vi "RTP_RTSP - Parse RTP header.vi"(7 "RTP Packet":string) -> (8 "RTP Header":T1)   [LabVIEW 2014]
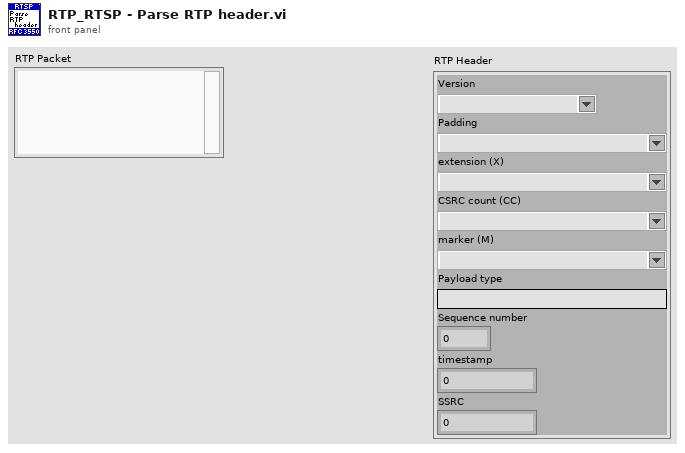
[diagram p1: front panel]
types:
  T1 = cluster{"Version":string, "Padding":string, "extension (X)":string, "CSRC count (CC)":string, "marker (M)":string, "Payload type":string, "Sequence number":u32, "timestamp":u32, "SSRC":u32}
  T2 = cluster{string, string, string, string, string, string, u32, u32, u32}
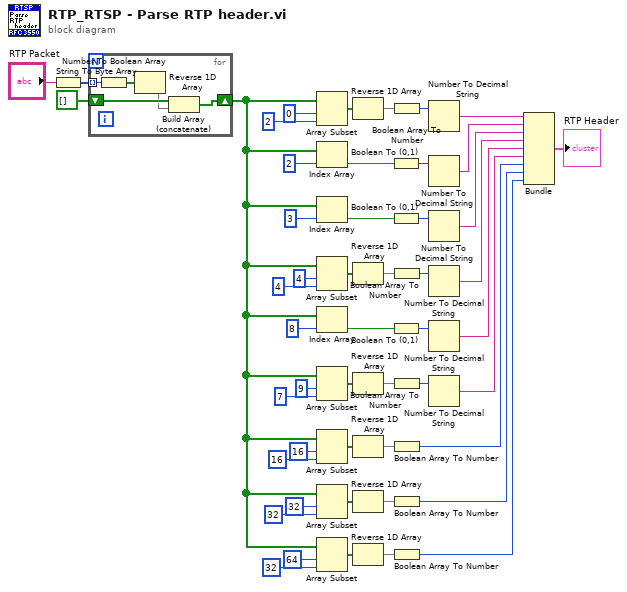
[diagram p0: block diagram]
diagram:
  n1 = String To Byte Array(string="RTP Packet") -> (unsigned byte array=w48:u8[])
  n2 = for {
    tunnel: w48 -> [w55] mode=indexing
    shift-right: [w52] -> w11
    shift-left: bool[] [] -> [w54]
    n3 = Number To Boolean Array(number=w55) -> (Boolean array=w53:bool[])
    n4 = Reverse 1D Array(array=w53) -> (reversed array=w51:bool[])
    n5 = Build Array (concatenate)(w54, w51) -> (w52:bool[])
  }
  n6 = Array Subset(array=w11, index=0, length=2) -> (w45:bool[])
  n7 = Index Array(array=w11, index=2) -> (element=w41:bool)
  n8 = Index Array(array=w11, index=3) -> (element=w38:bool)
  n9 = Array Subset(array=w11, index=4, length=4) -> (w34:bool[])
  n10 = Index Array(array=w11, index=8) -> (element=w30:bool)
  n11 = Array Subset(array=w11, index=9, length=7) -> (w20:bool[])
  n12 = Array Subset(array=w11, index=16, length=16) -> (w23:bool[])
  n13 = Array Subset(array=w11, index=32, length=32) -> (w17:bool[])
  n14 = Array Subset(array=w11, index=64, length=32) -> (w14:bool[])
  n15 = Reverse 1D Array(array=w45) -> (reversed array=w44:bool[])
  n16 = Reverse 1D Array(array=w34) -> (reversed array=w35:bool[])
  n17 = Reverse 1D Array(array=w20) -> (reversed array=w26:bool[])
  n18 = Reverse 1D Array(array=w23) -> (reversed array=w24:bool[])
  n19 = Reverse 1D Array(array=w17) -> (reversed array=w16:bool[])
  n20 = Reverse 1D Array(array=w14) -> (reversed array=w15:bool[])
  n21 = Boolean To (0,1)(Boolean=w41) -> (0, 1=w40:i16)
  n22 = Boolean To (0,1)(Boolean=w38) -> (0, 1=w39:i16)
  n23 = Boolean To (0,1)(Boolean=w30) -> (0, 1=w29:i16)
  n24 = Boolean Array To Number(Boolean array=w44) -> (number=w43:u32)
  n25 = Boolean Array To Number(Boolean array=w35) -> (number=w36:u32)
  n26 = Boolean Array To Number(Boolean array=w26) -> (number=w25:u32)
  n27 = Boolean Array To Number(Boolean array=w24) -> (number=w4:u32)
  n28 = Boolean Array To Number(Boolean array=w16) -> (number=w3:u32)
  n29 = Boolean Array To Number(Boolean array=w15) -> (number=w2:u32)
  n30 = Number To Decimal String(number=w43) -> (decimal integer string=w10:string)  [unwired: 1 in]
  n31 = Number To Decimal String(number=w40) -> (decimal integer string=w9:string)  [unwired: 1 in]
  n32 = Number To Decimal String(number=w39) -> (decimal integer string=w8:string)  [unwired: 1 in]
  n33 = Number To Decimal String(number=w36) -> (decimal integer string=w7:string)  [unwired: 1 in]
  n34 = Number To Decimal String(number=w29) -> (decimal integer string=w6:string)  [unwired: 1 in]
  n35 = Number To Decimal String(number=w25) -> (decimal integer string=w5:string)  [unwired: 1 in]
  n36 = Bundle(w10, w9, w8, w7, w6, w5, w4, w3, w2) -> (→"RTP Header":T2)  [unwired: 1 in]
